vi "Run Batch.vi"() -> ()   [LabVIEW 2010]
doc: "The purpose of this VI is to run a batch parameters file. The user should simply enter the path and filename of the batch parameters file and then click the \"Run Batch\" button. The \"Stop\" button can be used to end execution of the program. On the coding side, the program will read in the batch parameter file, which will typically be a tab-delimited text file (if it was made with the \"Test and Make Batch.vi\" program). The file is read into a 2-D array of strings and then a for-loop is used to strip out one row of the batch parameters array at a time. Each separate parameter is stripped out of that row, and then converted into the data type required by the \"MMB SubVI.vi\" program. The parameters are then sent to \"MMB SubVI.vi\", it executes, and then the next row from the 2-D string array is processed until all rows have been sent and executed."
uses:
  <vilib>/Utility/file.llb/Read From Spreadsheet File (string).vi
panel:
  in  "stop":bool
  in  "Run":bool
  in  "Batch":path=path "c:/Ed's Files/LabVIEW Files/My Code/Moving Message Board/Sample Batch Files/Batch.txt" caption="Batch Parameters File Path"
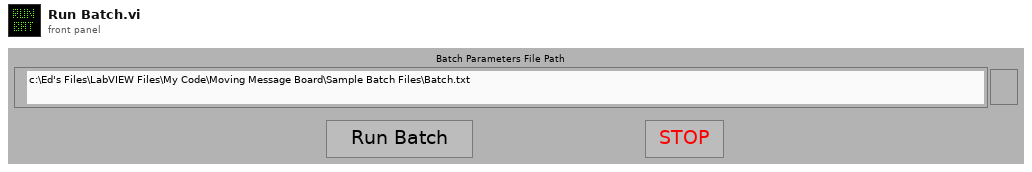
[diagram p1: front panel]
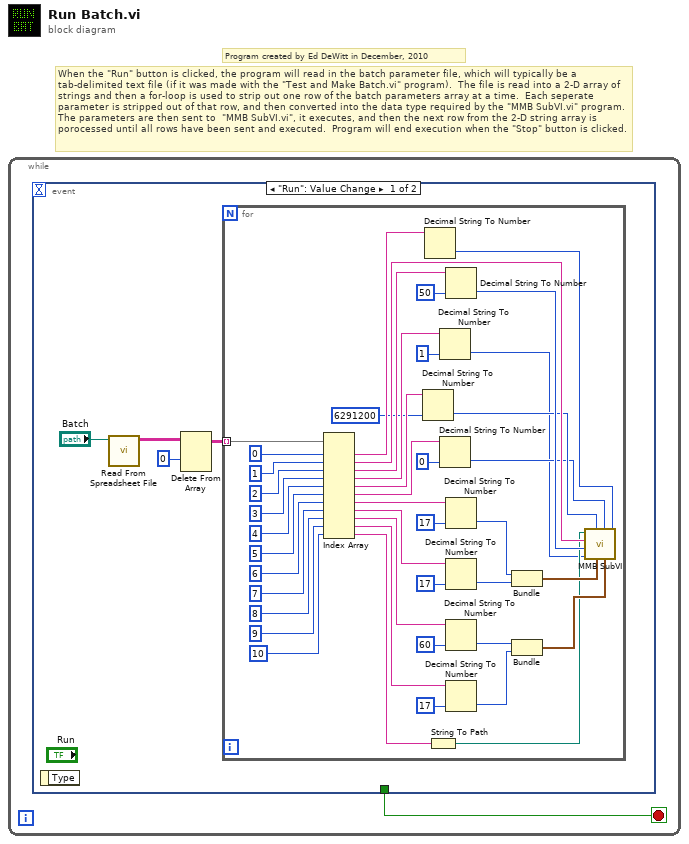
[diagram p0: block diagram]
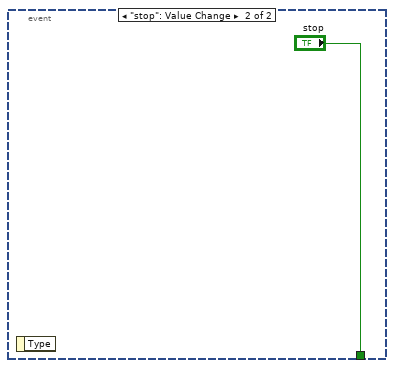
[diagram p2: hidden frame]
diagram:
  # "When the \"Run\" button is clicked, the program will read in the batch parameter file, which will typically be a tab-delimited text file (if it was made with the \"Test and Make Batch.vi\" program).  The file is read into a 2-D array of strings and then a for-loop is used to strip out one row of the batch parameters array at a time.  Each seperate parameter is stripped out of that row, and then converted into the data type required by the \"MMB SubVI.vi\" program.  The parameters are then sent to  \"MMB SubVI.vi\", it executes, and then the next row from the 2-D string array is porocessed until all rows have been sent and executed.  Program will end execution when the \"Stop\" button is clicked."
  # "Program created by Ed DeWitt in December, 2010"
  n1 = while {
    stop <- w1 stop-if-true
    n2 = event shown="[0] \"Run\": Value Change" {
      selector: _ -> [_ _]
      dyn-events: _ -> [_ _]
      timeout: _ -> [_ _]
      tunnel: [_ "stop"] -> w1
      event "Run": Value Change {
        n3 = event-data() -> ()  [unwired: 1 in, 1 out]
        n4 = call-poly <vilib>:"Read From Spreadsheet File.vi"("file path (dialog if empty)"="Batch") -> ("all rows"=w4:string[][])  [unwired: 6 in, 4 out]
        n5 = Delete From Array(array=w4, index (row)=0) -> (array with subset deleted=w2:string[][])  [unwired: 2 in, 1 out]
        n6 = for {
          tunnel: w2 -> [w48] mode=indexing
          n7 = Index Array(array=w48, index #1=0 ("index"), index #2=1 ("index"), index #3=2 ("index"), index #4=3 ("index"), index #5=4 ("index"), index #6=5 ("index"), index #7=6 ("index"), index #8=7 ("index"), index #9=8 ("index"), index #10=9 ("index"), index #11=10 ("index")) -> (element #1=w46:string, element #2=w44:string, element #3=w42:string, element #4=w39:string, element #5=w37:string, element #6=w34:string, element #7=w22:string, element #8=w20:string, element #9=w18:string, element #10=w16:string, element #11=w10:string)
          n8 = Decimal String To Number(string=w37, default (0L)=u32 6291200 ("default (0 I32)")) -> (number=w36:u32)  [unwired: 1 in, 1 out]
          n9 = Decimal String To Number(string=w46) -> (number=w6:i32)  [unwired: 2 in, 1 out]
          n10 = String To Path(string=w10) -> (path=w9:path)
          n11 = Decimal String To Number(string=w39, default (0L)=u64 1 ("default (0 I32)")) -> (number=w7:u64)  [unwired: 1 in, 1 out]
          n12 = Decimal String To Number(string=w34, default (0L)=u32 0 ("default (0 I32)")) -> (number=w33:u32)  [unwired: 1 in, 1 out]
          n13 = Decimal String To Number(string=w42, default (0L)=u32 50 ("default (0 I32)")) -> (number=w40:u32)  [unwired: 1 in, 1 out]
          n14 = Decimal String To Number(string=w22, default (0L)=u32 17 ("default (0 I32)")) -> (number=w29:u32)  [unwired: 1 in, 1 out]
          n15 = Decimal String To Number(string=w20, default (0L)=u32 17 ("default (0 I32)")) -> (number=w28:u32)  [unwired: 1 in, 1 out]
          n16 = Decimal String To Number(string=w18, default (0L)=u32 60 ("default (0 I32)")) -> (number=w26:u32)  [unwired: 1 in, 1 out]
          n17 = Decimal String To Number(string=w16, default (0L)=u32 17 ("default (0 I32)")) -> (number=w25:u32)  [unwired: 1 in, 1 out]
          n18 = Bundle(w29, w28) -> (w27:cluster{u32, u32})  [unwired: 1 in]
          n19 = Bundle(w26, w25) -> (w24:cluster{u32, u32})  [unwired: 1 in]
          n20 = call "MMB SubVI.vi"("Mode"=w6, "Array Size"=w24, "LED Off Color"=w33, "LED Size"=w27, "LED On Color"=w36, "Repeat/Hold"=w7, "Delay"=w40, "Message"=w44, "Config Path"=w9) -> ()  [unwired: 3 in]
        }
      }
      event "stop": Value Change {
        n21 = event-data() -> ()  [unwired: 1 in, 1 out]
      }
    }
  }
